vi "Convert String to Params.vi"(8 "error in (no error)":errorcluster, 11 "String In":string) -> (0 "error out":errorcluster, 3 "Param Out":T1={"Step Values"=[], "Only Execute When Test Running"=FALSE, "Reset Sequence When Test Starts"=TRUE, "Current Sequence ID"=0, "Total Iterations"=0, "Current Step Start Timestamp"=0.0, "Number of Sequence Steps"=0, "Num of Analog Channels"=0, "Num of Digital Channels"=0, "Delay Before Starting Sequence"=0.0, "Show UI"=FALSE, "Time Remaining"=0.0, "Test Running"=FALSE, "Pause Timestamp"=0.0, "Default Analog Values"=[], "Default Digital Values"=[]})   [LabVIEW 2024, in "Sequencer with Output Values.lvlib" / "Sequencer with Output Values.lvclass"]
uses:
  Sequencer with Output Values.lvclass
  Params.ctl
  Step Settings.ctl
  Global Strings.vi
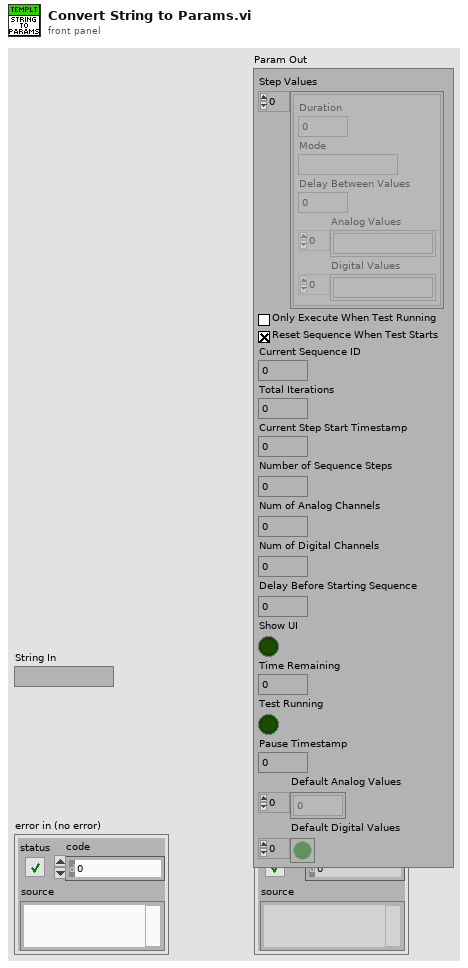
[diagram p1: front panel]
types:
  T1 = typedef "Sequencer with Output Values.lvlib/Sequencer with Output Values.lvclass/Params.ctl" = cluster{"Step Values":T2[], "Only Execute When Test Running":bool, "Reset Sequence When Test Starts":bool, "Current Sequence ID":u32, "Total Iterations":u32, "Current Step Start Timestamp":dbl, "Number of Sequence Steps":i32, "Num of Analog Channels":i32, "Num of Digital Channels":i32, "Delay Before Starting Sequence":dbl, "Show UI":bool, "Time Remaining":dbl, "Test Running":bool, "Pause Timestamp":dbl, "Default Analog Values":dbl[], "Default Digital Values":bool[]}
  T2 = typedef "Sequencer with Output Values.lvlib/Sequencer with Output Values.lvclass/Step Settings.ctl" = cluster{"Duration":dbl, "Mode":string, "Delay Between Values":dbl, "Analog Values":string[], "Digital Values":string[]}
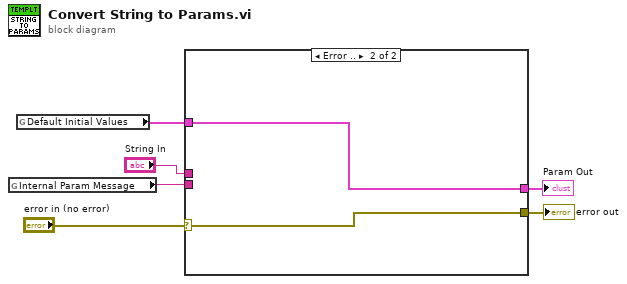
[diagram p0: block diagram]
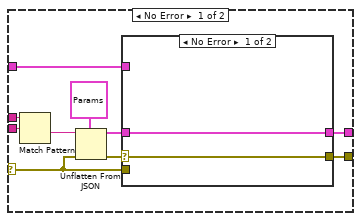
[diagram p2: hidden frame]
diagram:
  n1 = global read "Global Strings.vi" "Internal Param Message"() -> (w5:string)
  n2 = global read "Global Strings.vi" "Default Initial Values"() -> (w1:T1)
  n3 = case shown="Error .." "error in (no error)" {
    selector: "error in (no error)" -> [w8 w22]
    tunnel: "String In" -> [w14 _]
    tunnel: w5 -> [w13 _]
    tunnel: [w10 w21] -> w3
    tunnel: [w9 w22] -> w2
    tunnel: w1 -> [w7 w21]
    frame No Error {
      n4 = Match Pattern(string=w14, regular expression=w13) -> (after substring=w15:string)  [unwired: 1 in, 3 out]
      n5 = Unflatten From JSON(JSON string=w15, type and defaults=T1 {"Step Values"=[], "Only Execute When Test Running"=FALSE, "Reset Sequence When Test Starts"=TRUE, "Current Sequence ID"=0, "Total Iterations"=0, "Current Step Start Timestamp"=0.0, "Number of Sequence Steps"=0, "Num of Analog Channels"=0, "Num of Digital Channels"=0, "Delay Before Starting Sequence"=0.0, "Show UI"=FALSE, "Time Remaining"=0.0, "Test Running"=FALSE, "Pause Timestamp"=0.0, "Default Analog Values"=[], "Default Digital Values"=[]} ("cluster in"), error in (no error)=w8) -> (value=w11:T1, error out=w12:errorcluster)  [unwired: 4 in]
      n6 = case shown="No Error" w12 {
        selector: w12 -> [w17 _]
        tunnel: w11 -> [w18 _]
        tunnel: [w18 w19] -> w10
        tunnel: [w17 w20] -> w9
        tunnel: w8 -> [_ w20]
        tunnel: w7 -> [_ w19]
        frame No Error {
        }
        frame Error {
        }
      }
    }
    frame Error {
    }
  }
  "error out" <- w2
  "Param Out" <- w3
